vi "Cryo-Con Get Parameters.vi"(8 "error in (no error)":errorcluster, 10 "Initial String":string, 11 "VISA Resource Name":refnum<visa-resource-name>) -> (0 "error out":errorcluster, 2 "Parameters":string, 3 "Data titles":string[](array[string])=["Neocer_T (K)"], 5 "VISA Resource Name out":refnum<visa-resource-name>)   [LabVIEW 2015]
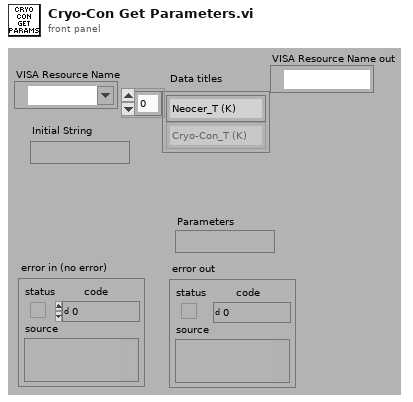
[diagram p1: front panel]
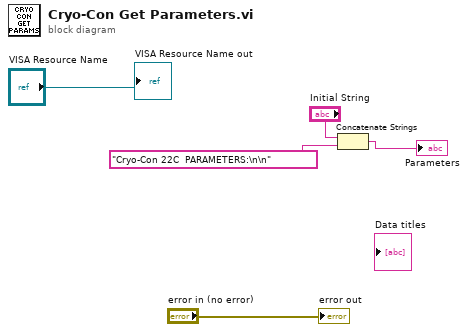
[diagram p0: block diagram]
diagram:
  n1 = Concatenate Strings("Initial String", "Cryo-Con 22C  PARAMETERS:\n\n") -> (→"Parameters":string)
  "error out" <- "error in (no error)"
  "VISA Resource Name out" <- "VISA Resource Name"
